vi "MotionMetricAll.vi"() -> ()   [LabVIEW 2017]
uses:
  <vilib>/Utility/file.llb/Write To Spreadsheet File (string).vi
  <vilib>/Utility/file.llb/Write To Spreadsheet File (DBL).vi
panel:
  out "Horizontal Progress Bar":u8(slide) scale=0.0..49.0
  out "Total Video Segments to Stabilize":dbl
  # "This VI stabilizes all AVI videos in the selected folder. The user is prompted to select the folder after which they are asked to choose the region to be stabilized for each video. The program will then run automously to stabilize all the videos."
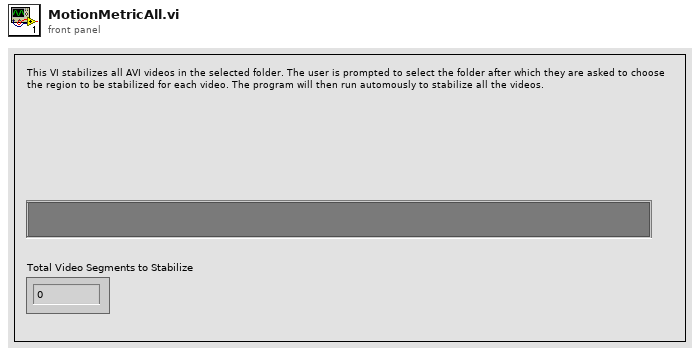
[diagram p1: front panel]
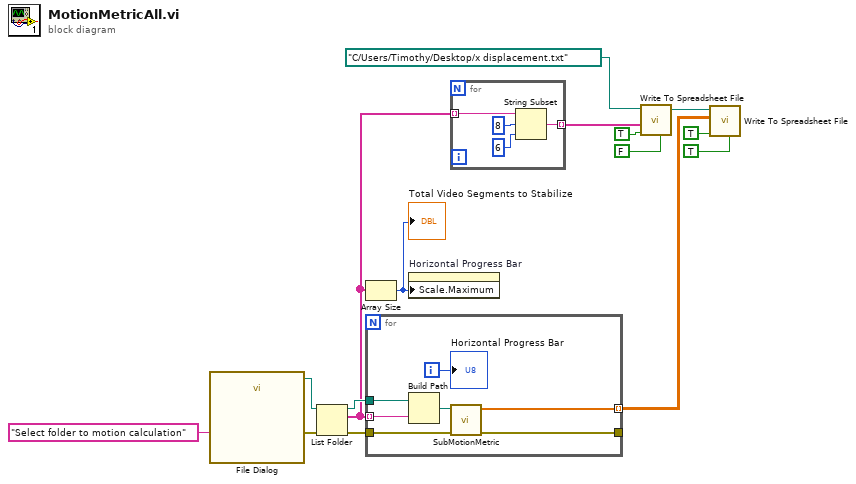
[diagram p0: block diagram]
diagram:
  n1 = call "File Dialog"("prompt"="Select folder to motion calculation") -> ("selected path"=w14:path, "error out"=w13:errorcluster)  [unwired: 11 in, 2 out]
  n2 = List Folder(path=w14, error in=w13) -> (path out=w12:path, filenames=w2:string[], error out=w11:errorcluster)  [unwired: 2 in, 1 out]
  n3 = Array Size(array=w2) -> (size(s)=w10:i32)
  "Total Video Segments to Stabilize" <- w10
  n4 = for {
    tunnel: w12 -> [w22]
    tunnel: w2 -> [w21] mode=indexing
    tunnel: w11 -> [w19]
    tunnel: [w17] -> w1 mode=indexing
    tunnel: [w16] -> _
    i -> [w18]
    n5 = Build Path(base path=w22, name or relative path=w21) -> (appended path=w20:path)
    n6 = call "SubMotionMetric.vi"("error in (no error)"=w19, "AVI Path"=w20) -> ("error out"=w16:errorcluster, "x displacement"=w17:sgl[])  [unwired: 6 in, 2 out]
    "Horizontal Progress Bar" <- w18
  }
  n7 = property on="Horizontal Progress Bar" class="Slide (strict)"("Scale.Maximum"=w10) -> ()  [unwired: 2 in, 2 out]
  n8 = for {
    tunnel: w2 -> [w26] mode=indexing
    tunnel: [w23] -> w3 mode=indexing
    n9 = String Subset(string=w26, offset (0)=8, length (rest)=6 ("length (rest)")) -> (substring=w23:string)
  }
  n10 = call-poly <vilib>:"Write To Spreadsheet File.vi"("transpose? (no:F)"=FALSE, "append to file? (new file:F)"=TRUE, "1D data"=w3, "file path (dialog if empty)"=path "C:/Users/Timothy/Desktop/x displacement.txt") -> ("new file path (Not A Path if cancelled)"=w4:path)  [unwired: 4 in]
  n11 = call-poly <vilib>:"Write To Spreadsheet File.vi"("transpose? (no:F)"=TRUE, "append to file? (new file:F)"=TRUE, "2D data"=w1, "file path (dialog if empty)"=w4) -> ()  [unwired: 4 in, 1 out]
